vi "SimpleConnectWithPublishAndSubscribe.vi"() -> ()   [LabVIEW 2016, in "AWS_IoT.lvlib"]
uses:
  AWS_IoT.lvlib
  MQTT/Controls/QoS.ctl
  MQTT/Controls/Retain_Flag.ctl
  MQTT/Controls/DUP_Flag.ctl
  Controls/certs.ctl
  MQTT/Controls/Connection_Return_Codes.ctl
  MQTT/Controls/ConnectMeta.ctl
  MQTT/Controls/Will_Info.ctl
  MQTT/Controls/MessageType.ctl
  MQTT/Controls/Connect_Flags.ctl
panel:
  out "delta t ms":u32
  in  "Stop Reading":bool
  out "error out 2":errorcluster
  out "Messages":T2(array[cluster])
  out "msg ct":i32
  in  "Subscription Info Array":cluster{"Topic":string, "QoS":T3}[](array[cluster])=[{"Topic"="testtopic/LVMQTT", "QoS"=enum."At most once"}]
  out "Granted QoS Levels":T3[](array[typedef])
  in  "Will Info":T4={"Will message"="Last Will", "Will Topic"="Will Topic"}
  in  "Connect Meta":T5={"Retain"=TRUE, "DUP"=FALSE, "Keep Alive (sec)"=60, "QoS"=enum."At most once"}
  out "Connection Status":T8=enum."Connection refused: not authorized"
  in  "cert path":T9={"client cert file"=path "", "CA file"=path "", "client key file"=path ""}
  in  "Publish Meta":cluster{"QoS":T3, "Retain":T6, "DUP":T7}
  in  "Topic":string="testtopic/LVMQTT"
  in  "error in (no error)":errorcluster
  in  "Client ID":string="LabVIEW_MQTT_Client"
  out "error out":errorcluster
  in  "MQTT Broker":cluster{"address (IP)":string, "port":u16}={"address (IP)"="a28e3t2sj3ekjh.iot.us-west-2.amazonaws.com", "port"=8883}
  in  "Message ID":u16=20
  in  "Stop Publishing":bool
  out "Message published":string
  out "Message ID (acknowledged)":u16=10
  out "Acknowledged":bool
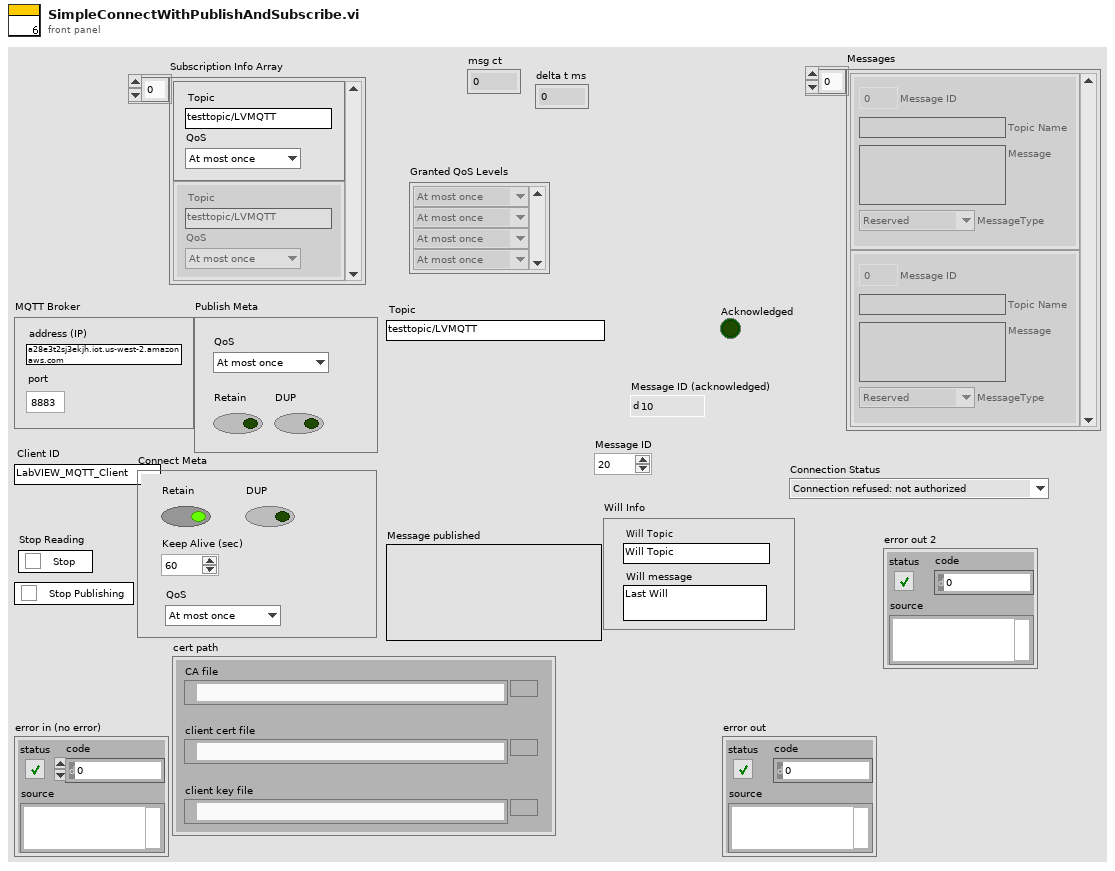
[diagram p1: front panel]
types:
  T1 = typedef "AWS_IoT.lvlib/MessageType.ctl" = enum32{"Reserved", "CONNECT", "CONNACK", "PUBLISH", "PUBACK", "PUBREC", "PUBREL", "PUBCOMP", "SUBSCRIBE", "SUBACK", "UNSUBSCRIBE", "UNSUBACK", "PINGREQ", "PINGRESP", "DISCONNECT", "Reserved2"}
  T2 = cluster{"Message ID":u16, "Topic Name":string, "Message ":string, "MessageType":T1}[]
  T3 = typedef "AWS_IoT.lvlib/QoS.ctl" = enum8{"At most once", "At least once", "Exactly once", "Reserved"}
  T4 = typedef "AWS_IoT.lvlib/Will_Info.ctl" = cluster{"Will message":string, "Will Topic":string}
  T5 = typedef "AWS_IoT.lvlib/ConnectMeta.ctl" = cluster{"Retain":T6, "DUP":T7, "Keep Alive (sec)":u16, "QoS":T3}
  T6 = typedef "AWS_IoT.lvlib/Retain_Flag.ctl" = bool
  T7 = typedef "AWS_IoT.lvlib/DUP_Flag.ctl" = bool
  T8 = typedef "AWS_IoT.lvlib/Connection_Return_Codes.ctl" = enum16{"Connection accepted", "Connection refused: unacceptable protocol version", "Connection refused: identifier rejected", "Connection refused: Server unavailable", "Connection refused: bad user name or password", "Connection refused: not authorized"}
  T9 = typedef "AWS_IoT.lvlib/certs.ctl" = cluster{"client cert file":path, "CA file":path, "client key file":path}
  T10 = cluster{"Message ID":u16, "Topic Name":string, "Message":string, "MessageType":T1}
  T11 = typedef "AWS_IoT.lvlib/Connect_Flags.ctl" = cluster{"user name":bool, "password":bool, "will retain":bool, "will flag":bool, "clean session":bool, "reserved":bool, "will QoS":T3}
  T12 = typedef "AWS_IoT.lvlib/SSL_Connection.ctl" = cluster{"connection ID":refnum<k5>, "TLS":cluster{"CXT ptr":i32, "SSL ptr":i32, "Socket ptr":i32}, "NIssleay library path":path, "server url":string}
  T13 = cluster{"Message ID":u16, "Topic Name":string, "Message":string, "MessageType":T1}[]
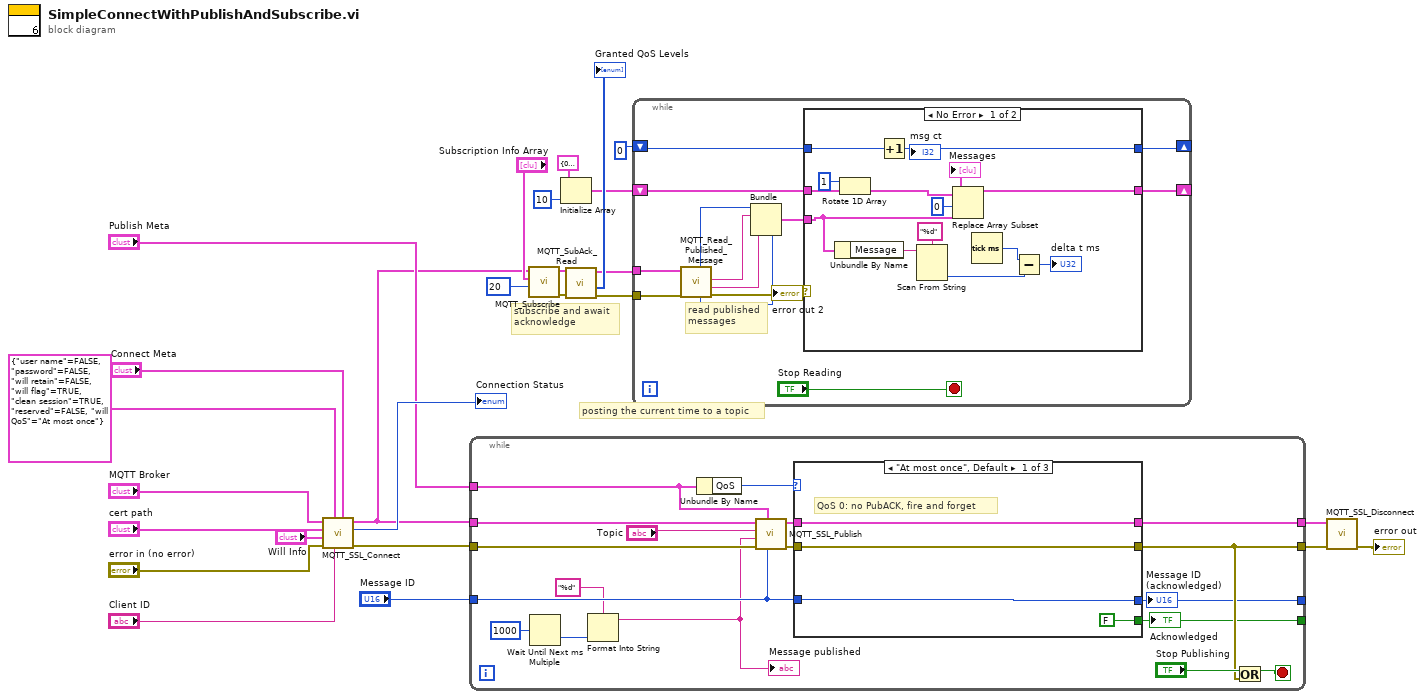
[diagram p0: block diagram]
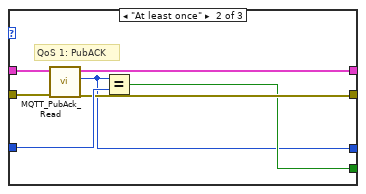
[diagram p3: hidden frame]
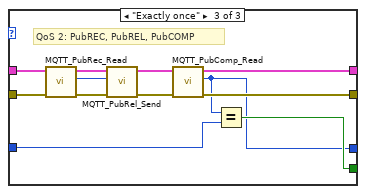
[diagram p4: hidden frame]
diagram:
  # "subscribe and await\nacknowledge"
  # "posting the current time to a topic"
  n1 = call "MQTT_SSL_Connect.vi"("Connect Meta"="Connect Meta", "Client ID"="Client ID", "Connect Flags"=T11 {"user name"=FALSE, "password"=FALSE, "will retain"=FALSE, "will flag"=TRUE, "clean session"=TRUE, "reserved"=FALSE, "will QoS"=enum."At most once"}, "error in (no error)"="error in (no error)", "Will Info"="Will Info", "cert path"="cert path", "MQTT Broker"="MQTT Broker") -> ("error out"=w26:errorcluster, "Connection Status"=→"Connection Status":T8, "SSL_Connection"=w1:T12)  [unwired: 2 in]
  n2 = while {
    tunnel: w1 -> [w31]
    tunnel: "Publish Meta" -> [w43]
    tunnel: [w39] -> w22
    tunnel: "Message ID" -> [w38]
    tunnel: [w33] -> _
    tunnel: [w32] -> _
    tunnel: w26 -> [w44]
    tunnel: [w35] -> w21
    stop <- w36 stop-if-true
    n3 = Wait Until Next ms Multiple(millisecond multiple=u32 1000) -> (millisecond timer value=w29:u32)
    n4 = Format Into String(format string="%d", w29) -> (resulting string=w27:string)  [unwired: 2 in, 1 out]
    "Message published" <- w27
    n5 = Unbundle By Name(w43) -> ("QoS"=w42:T3)
    n6 = call "MQTT_SSL_Publish.vi"("Message ID"=w38, "Publish Meta"=w43, "error in (no error)"=w44, "Message to be published"=w27, "Topic"="Topic", "SSL_Connection"=w31) -> ("error out"=w41:errorcluster, "SSL_Connection"=w40:T12)  [unwired: 4 in]
    n7 = case shown="\"At most once\", Default" w42 {
      tunnel: w41 -> [w47 w54 w66]
      tunnel: w40 -> [w48 w55 w67]
      tunnel: [w47 w52 w59] -> w35
      tunnel: [w48 w51 w60] -> w39
      tunnel: w38 -> [w45 w53 w65]
      tunnel: [FALSE w50 w61] -> w33
      tunnel: [w45 w49 w58] -> w32
      frame "At most once", Default {
        # "QoS 0: no PubACK, fire and forget"
      }
      frame "At least once" {
        # "QoS 1: PubACK"
        n8 = call "MQTT_PubAck_Read.vi"("error in (no error)"=w54, "SSL_Connection"=w55) -> ("error out"=w52:errorcluster, "Message ID"=w49:u16, "SSL_Connection"=w51:T12)  [unwired: 7 in]
        n9 = Equal?(x=w49, y=w53) -> (x = y?=w50:bool)
      }
      frame "Exactly once" {
        # "QoS 2: PubREC, PubREL, PubCOMP"
        n10 = call "MQTT_PubRec_Read.vi"("error in (no error)"=w66, "SSL_Connection"=w67) -> ("error out"=w64:errorcluster, "Message ID"=w62:u16, "SSL_Connection"=w63:T12)  [unwired: 7 in]
        n11 = call "MQTT_PubRel_Send.vi"("error in (no error)"=w64, "Message ID"=w62, "SSL_Connection"=w63) -> ("error out"=w56:errorcluster, "SSL_Connection"=w57:T12)  [unwired: 6 in, 1 out]
        n12 = call "MQTT_PubComp_Read.vi"("error in (no error)"=w56, "SSL_Connection"=w57) -> ("error out"=w59:errorcluster, "Message ID"=w58:u16, "SSL_Connection"=w60:T12)  [unwired: 7 in]
        n13 = Equal?(x=w58, y=w65) -> (x = y?=w61:bool)
      }
    }
    "Message ID (acknowledged)" <- w32
    "Acknowledged" <- w33
    n14 = Or(x="Stop Publishing", y=w35) -> (x .or. y?=w36:bool)
  }
  n15 = call "MQTT_Subscribe.vi"("Message ID"=u16 20, "Subscription Info Array"="Subscription Info Array", "SSL_Connection"=w1) -> ("error out"=w9:errorcluster, "SSL_Connection"=w6:T12)  [unwired: 7 in]
  n16 = Initialize Array(T10 {"Message ID"=0, "Topic Name"="", "Message"="", "MessageType"=enum."Reserved"}, 10 ("dimension size")) -> (w3:T13)
  n17 = call "MQTT_SubAck_Read.vi"("error in (no error)"=w9, "SSL_Connection"=w6) -> ("error out"=w11:errorcluster, "Granted QoS Levels"=→"Granted QoS Levels":T3[], "SSL_Connection 2"=w10:T12)  [unwired: 7 in]
  n18 = while {
    shift-right: [w78] -> _
    shift-left: w3 -> [w80]
    tunnel: w11 -> [w76]
    tunnel: w10 -> [w77]
    shift-right: [w69] -> _
    shift-left: 0 -> [w70]
    stop <- "Stop Reading" stop-if-true
    # "read published\nmessages"
    n19 = call "MQTT_Read_Published_Message.vi"("error in (no error)"=w76, "SSL_Connection"=w77) -> ("error out"=w71:errorcluster, "Message"=w68:string, "Topic Name"=w75:string, "MessageType"=w73:T1, "Message ID"=w74:u16)  [unwired: 4 in, 1 out]
    "error out 2" <- w71
    n20 = Bundle("Message ID"=w74, "Topic Name"=w75, "Message"=w68, "MessageType"=w73) -> (w79:T10)  [unwired: 1 in]
    n21 = case shown="No Error" w71 {
      tunnel: w80 -> [w93 w95]
      tunnel: w79 -> [w86 _]
      tunnel: [w92 w95] -> w78
      tunnel: w70 -> [w88 w94]
      tunnel: [w87 w94] -> w69
      frame No Error {
        n22 = Unbundle By Name(w86) -> ("Message"=w84:string)
        n23 = Rotate 1D Array(1:w93, 2:1 ("n")) -> (0:w90:T13)
        n24 = Increment(x=w88) -> (x+1=w87:i32)
        "msg ct" <- w87
        n25 = Scan From String(format string="%d", input string=w84) -> (output 1=w82:i32)  [unwired: 3 in, 3 out]
        n26 = Replace Array Subset(array=w90, new element=w86, index=0) -> (w92:T13)
        "Messages" <- w92
        n27 = Tick Count (ms)() -> (millisecond timer value=w83:u32)
        n28 = Subtract(x=w83, y=w82) -> (x-y=→"delta t ms":u32)
      }
      frame Error {
      }
    }
  }
  n29 = call "MQTT_SSL_Disconnect.vi"("error in (no error)"=w21, "SSL_Connection"=w22) -> ("error out"=→"error out":errorcluster)  [unwired: 9 in]
